vi "Configure Display Cycle in Op Screen.vi"(8 "error in (no error)":errorcluster, 9 "Display Cycle in Op Screen (1)":i16=1 min=0 max=1 step=1, 11 "VISA resource name":refnum<visa-resource-name>) -> (0 "error out":errorcluster, 3 "VISA resource name out":refnum<visa-resource-name>)   [LabVIEW 2010, in "Temptronic TP04300.lvlib"]
doc: "This VI configures the Operator Screen for TP04300 instrument.\n\n<b>Display Cycle in Operator Screen Flag</b> - 0 to hide Cycle Controls \nand 1 - to diplay them in the Operator Screen.\n\nDefault Value: 1\nValid Range: 0 - 1"
uses:
  Temptronic TP04300.lvlib
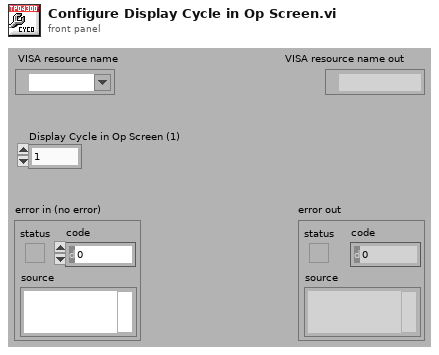
[diagram p1: front panel]
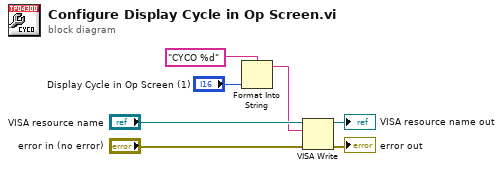
[diagram p0: block diagram]
diagram:
  n1 = Format Into String(format string="CYCO %d", "Display Cycle in Op Screen (1)") -> (resulting string=w3:string)  [unwired: 2 in, 1 out]
  n2 = VISA Write(VISA resource name="VISA resource name", write buffer=w3, error in (no error)="error in (no error)") -> (VISA resource name out=→"VISA resource name out":refnum<visa-resource-name>, error out=→"error out":errorcluster)  [unwired: 1 out]
